vi "comandoLockin530.vi"(8 "error in":errorcluster, 10 "Comando":string="AP;") -> (0 "error out":errorcluster, 1 "Fase":dbl)   [LabVIEW 2018]
uses:
  <vilib>/Instr/_visa.llb/VISA Configure Serial Port (Instr).vi
panel:
  out "X":dbl
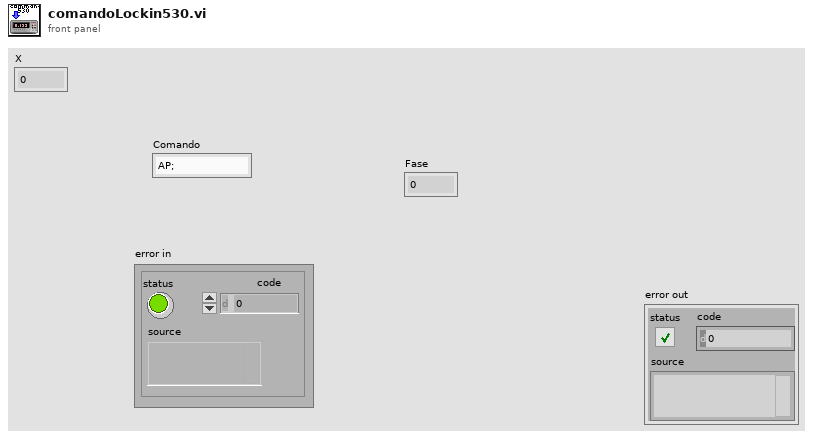
[diagram p1: front panel]
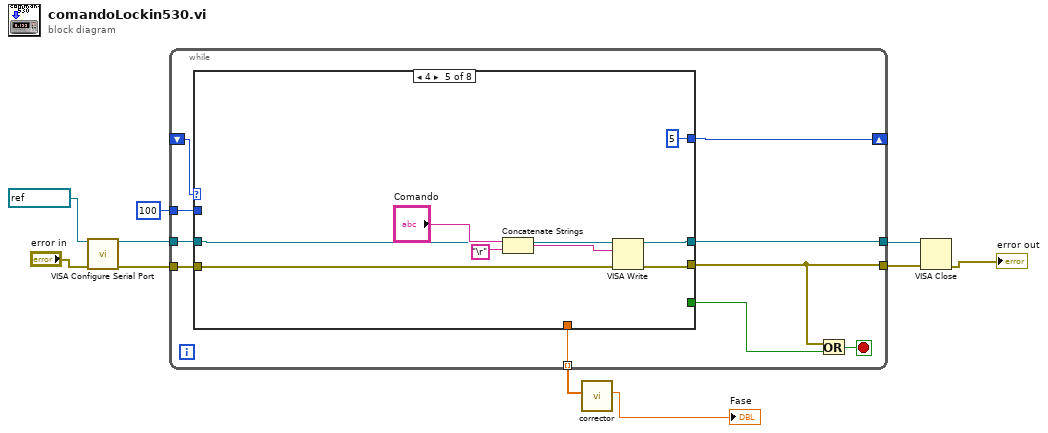
[diagram p0: block diagram]
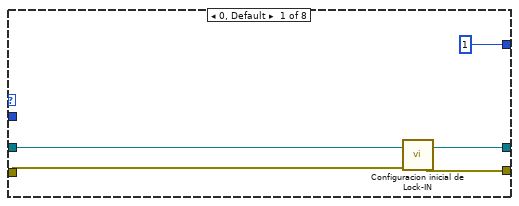
[diagram p2: hidden frame]
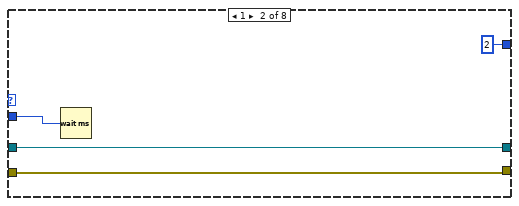
[diagram p3: hidden frame]
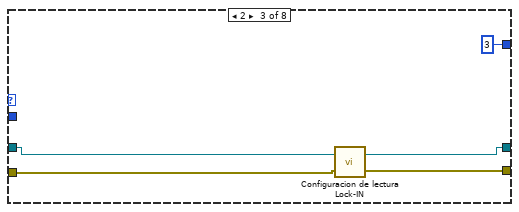
[diagram p4: hidden frame]
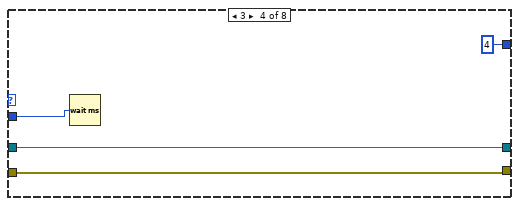
[diagram p5: hidden frame]
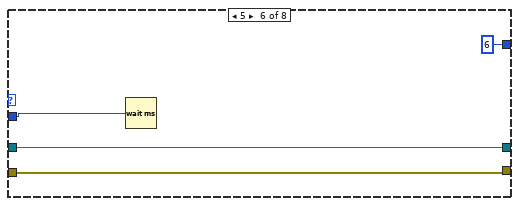
[diagram p6: hidden frame]
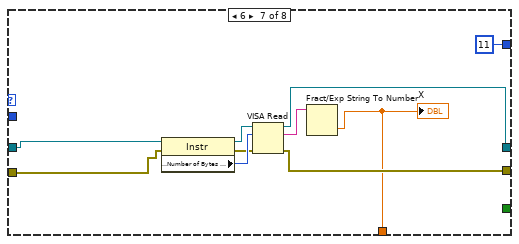
[diagram p7: hidden frame]
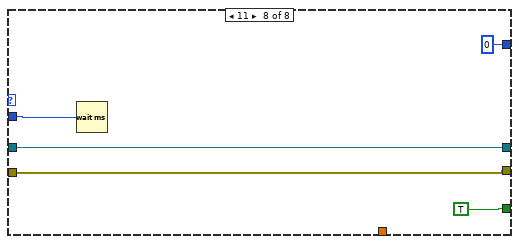
[diagram p8: hidden frame]
diagram:
  n1 = call-poly "VISA Configure Serial Port"("VISA resource name"=refnum<visa-resource-name> "COM4", "error in (no error)"="error in") -> ("VISA resource name out"=w8:refnum<visa-resource-name>, "error out"=w7:errorcluster)  [unwired: 12 in]
  n2 = while {
    shift-right: [w16] -> _
    shift-left: _ -> [w20]
    tunnel: w8 -> [w18]
    tunnel: w7 -> [w17]
    tunnel: 100 -> [w15]
    tunnel: [w14] -> w1
    tunnel: [w13] -> w3
    tunnel: [w11] -> w5 mode=indexing
    stop <- w19 stop-if-true
    n3 = case shown="4" w20 {
      tunnel: w18 -> [w25 w27 w34 w37 w42 w49 w56 w64]
      tunnel: w17 -> [w24 w26 w33 w36 w41 w48 w55 w63]
      tunnel: [1 2 3 4 5 6 11 0] -> w16
      tunnel: w15 -> [_ w29 _ w38 _ w50 _ w62]
      tunnel: [w22 w27 w32 w37 w43 w49 w54 w64] -> w14
      tunnel: [w21 w26 w31 w36 w40 w48 w53 w63] -> w13
      tunnel: [_ _ _ _ _ _ _ TRUE] -> w12
      tunnel: [_ _ _ _ _ _ w51 _] -> w11
      frame 0, Default {
        n4 = call "Configuracion inicial de Lock-IN.vi"("error in (no error)"=w24, "VISA resource name"=w25) -> ("error out"=w21:errorcluster, "VISA resource name out"=w22:refnum<visa-resource-name>)
      }
      frame 1 {
        n5 = Wait (ms)(milliseconds to wait=w29) -> ()  [unwired: 1 out]
      }
      frame 2 {
        n6 = call "Configuracion de lectura Lock-IN.vi"("error in (no error)"=w33, "VISA resource name"=w34) -> ("error out"=w31:errorcluster, "VISA resource name out"=w32:refnum<visa-resource-name>)
      }
      frame 3 {
        n7 = Wait (ms)(milliseconds to wait=w38) -> ()  [unwired: 1 out]
      }
      frame 4 {
        n8 = Concatenate Strings("Comando", "\r") -> (w44:string)
        n9 = VISA Write(VISA resource name=w42, write buffer=w44, error in (no error)=w41) -> (VISA resource name out=w43:refnum<visa-resource-name>, error out=w40:errorcluster)  [unwired: 1 out]
      }
      frame 5 {
        n10 = Wait (ms)(milliseconds to wait=w50) -> ()  [unwired: 1 out]
      }
      frame 6 {
        n11 = property class="Instr"(reference=w56, error in=w55) -> (reference out=w60:refnum<visa-resource-name>, error out=w58:errorcluster, "Serial Settings:Number of Bytes at Serial Port"=w59:u32)
        n12 = VISA Read(VISA resource name=w60, byte count=w59, error in (no error)=w58) -> (VISA resource name out=w54:refnum<visa-resource-name>, read buffer=w57:string, error out=w53:errorcluster)  [unwired: 1 out]
        n13 = Fract/Exp String To Number(string=w57) -> (number=w51:dbl)  [unwired: 3 in, 1 out]
        "X" <- w51
      }
      frame 11 {
        n14 = Wait (ms)(milliseconds to wait=w62) -> ()  [unwired: 1 out]
      }
    }
    n15 = Or(x=w13, y=w12) -> (x .or. y?=w19:bool)
  }
  n16 = call "corrector.vi"("Array"=w5) -> ("valor salida"=→"Fase":dbl)  [unwired: 10 in]
  n17 = VISA Close(VISA resource name=w1, error in (no error)=w3) -> (error out=→"error out":errorcluster)
